vi "FT10_Fornax MonopolarCommand.vi"(0 "EnergyChannelID":T6, 1 "Serial Number":T1, 5 "CutMode":T5, 7 "CoagMode":T4, 9 "CutPowerCommand":T3, 11 "CoagPowerCommand":T2) -> (4 "JSON Command":string)   [LabVIEW 2024]
uses:
  Controls/Control_Fornax Set Monopolar Command - Energy Channel ID Enum.ctl
  Controls/Control_Fornax Set Monopolar Command - Cut Mode Enum.ctl
  Controls/Control_Fornax Set Monopolar Command - Coag Mode Enum.ctl
  Controls/Control_Fornax Set Monopolar Command - Cut Power Command Enum.ctl
  Controls/Control_Fornax Set Monopolar Command - Coag Power Command Enum.ctl
  Controls/Control_Fornax Set Monopolar Command - Serial Number String.ctl
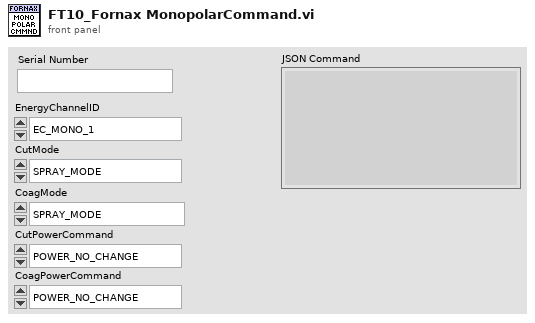
[diagram p1: front panel]
types:
  T1 = typedef "Control_Fornax Set Monopolar Command - Serial Number String.ctl" = string
  T2 = typedef "Control_Fornax Set Monopolar Command - Coag Power Command Enum.ctl" = enum16{"POWER_NO_CHANGE", "POWER_INCREASE", "POWER_DECREASE", "POWER_INCREASE_REPEAT", "POWER_DECREASE_REPEAT"}
  T3 = typedef "Control_Fornax Set Monopolar Command - Cut Power Command Enum.ctl" = enum16{"POWER_NO_CHANGE", "POWER_INCREASE", "POWER_DECREASE", "POWER_INCREASE_REPEAT", "POWER_DECREASE_REPEAT"}
  T4 = typedef "Control_Fornax Set Monopolar Command - Coag Mode Enum.ctl" = enum16{"SPRAY_MODE", "CUT_MODE", "BLEND_MODE", "FULGERATE_MODE", "BEPOLAR_MODE", "VESSEL_SEALING_MODE", "VALLEYLAB_MODE", "BIPOLAR_RESECTION_CUT_MODE", "BIPOLAR_RESECTION_COAG_MODE", "AUTOBIPOLAR_MODE", "VIPER_HLA", "SOFT_COAG_MODE", "NUM_ENERGY_MODES"}
  T5 = typedef "Control_Fornax Set Monopolar Command - Cut Mode Enum.ctl" = enum16{"SPRAY_MODE", "CUT_MODE", "BLEND_MODE", "FULGERATE_MODE", "BIPOLAR_MODE", "VESSEL_SEALING_MODE", "VALLEYLAB_MODE", "BIPOLAR_RESECTION_CUT_MODE", "BIPOLAR_RESECTION_COAG_MODE", "AUTOBIPOLAR_MODE", "VIPER_HLA", "SOFT_COAG_MODE", "NUM_ENERGY_MODES"}
  T6 = typedef "Control_Fornax Set Monopolar Command - Energy Channel ID Enum.ctl" = enum16{"EC_MONO_1", "EC_BIPOLAR", "EC_MONO_2", "EC_ADVANCED", "NUM_ENERGY_CHANNELS", "EC_NOT_USED"}
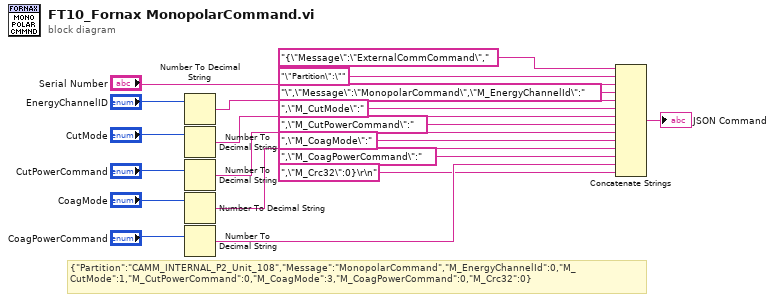
[diagram p0: block diagram]
diagram:
  # "{\"Partition\":\"CAMM_INTERNAL_P2_Unit_108\",\"Message\":\"MonopolarCommand\",\"M_EnergyChannelId\":0,\"M_CutMode\":1,\"M_CutPowerCommand\":0,\"M_CoagMode\":3,\"M_CoagPowerCommand\":0,\"M_Crc32\":0}"
  n1 = Number To Decimal String(number="EnergyChannelID") -> (decimal integer string=w10:string)  [unwired: 1 in]
  n2 = Number To Decimal String(number="CutMode") -> (decimal integer string=w12:string)  [unwired: 1 in]
  n3 = Number To Decimal String(number="CutPowerCommand") -> (decimal integer string=w15:string)  [unwired: 1 in]
  n4 = Number To Decimal String(number="CoagMode") -> (decimal integer string=w17:string)  [unwired: 1 in]
  n5 = Number To Decimal String(number="CoagPowerCommand") -> (decimal integer string=w20:string)  [unwired: 1 in]
  n6 = Concatenate Strings("{\"Message\":\"ExternalCommCommand\",", "\"Partition\":\"", "Serial Number", "\",\"Message\":\"MonopolarCommand\",\"M_EnergyChannelId\":" ("string"), w10, ",\"M_CutMode\":" ("string"), w12, ",\"M_CutPowerCommand\":" ("string"), w15, ",\"M_CoagMode\":" ("string"), w17, ",\"M_CoagPowerCommand\":" ("string"), w20, ",\"M_Crc32\":0}\r\n" ("string")) -> (→"JSON Command":string)
